vi "BootCommand.vi"(0 "VISA resource name":refnum<visa-resource-name>="COM1", 1 "error in (no error)":errorcluster {"code" format="%.0x"}) -> (2 "VISA resource name Out":refnum<visa-resource-name>, 3 "Receive_buffer":u8[](array[numeric]), 4 "error out":errorcluster)   [LabVIEW 2014]
panel:
  out "Read Count":u32
  out "Write Count":u32
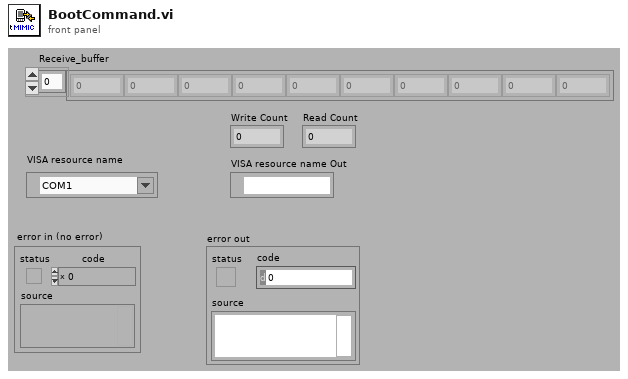
[diagram p1: front panel]
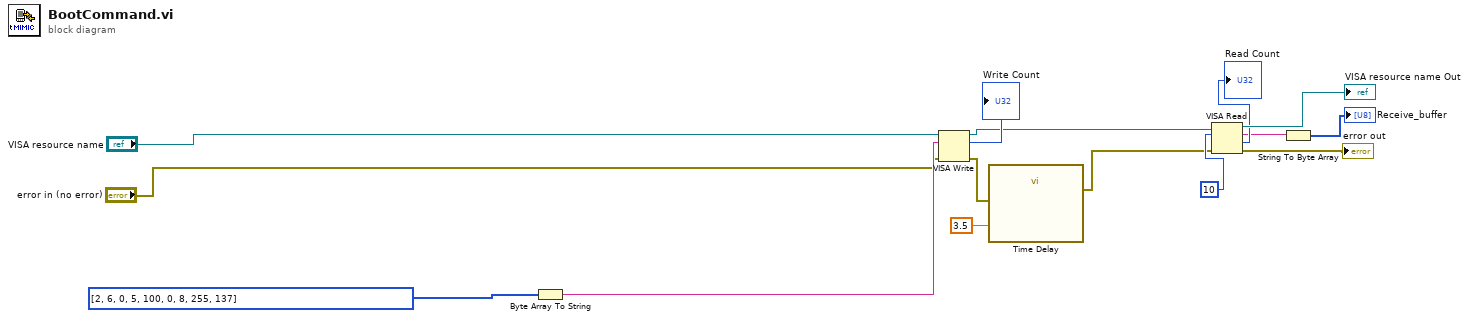
[diagram p0: block diagram]
diagram:
  n1 = Byte Array To String(unsigned byte array=u8[] [2, 6, 0, 5, 100, 0, 8, 255, 137] ("Command array")) -> (string=w13:string)
  n2 = VISA Write(VISA resource name="VISA resource name", write buffer=w13, error in (no error)="error in (no error)") -> (VISA resource name out=w4:refnum<visa-resource-name>, return count=→"Write Count":u32, error out=w5:errorcluster)
  n3 = call "Time Delay"("error in (no error)"=w5, "Delay Time (s)"=3.5) -> ("error out"=w3:errorcluster)  [unwired: 9 in]
  n4 = VISA Read(VISA resource name=w4, byte count=u32 10, error in (no error)=w3) -> (VISA resource name out=→"VISA resource name Out":refnum<visa-resource-name>, read buffer=w8:string, return count=→"Read Count":u32, error out=→"error out":errorcluster)
  n5 = String To Byte Array(string=w8) -> (unsigned byte array=→"Receive_buffer":u8[])
